vi "Template Tool Global.vi"() -> ()   [LabVIEW 2020, in "Template Tool.lvlib"]
uses:
  Template Tool.lvlib
panel:
  in  "CD support lvproj name":string
  in  "CD lvproj name":string
  in  "CD name":string
  in  "xml name":string
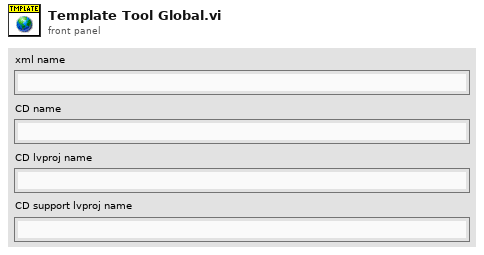
[diagram p1: front panel]
diagram:
